vi "getEvents.vi"(8 "error in (no error)":errorcluster, 11 "ScriptEdEvents in":refnum<class "ScriptEdEvents.lvclass">) -> (0 "error out":errorcluster, 1 "eventsToScriptEd":T1, 2 "ScriptEvent":refnum<user-event>, 3 "ScriptEdEvents out":refnum<class "ScriptEdEvents.lvclass">)   [LabVIEW 2009, in "Views.lvlib" / "ScriptEditor.lvlib" / "ScriptEdEvents.lvclass"]
uses:
  ScriptEdEvents.lvclass
  ScriptEdEvents.lvclass/ScriptEdEvents.ctl
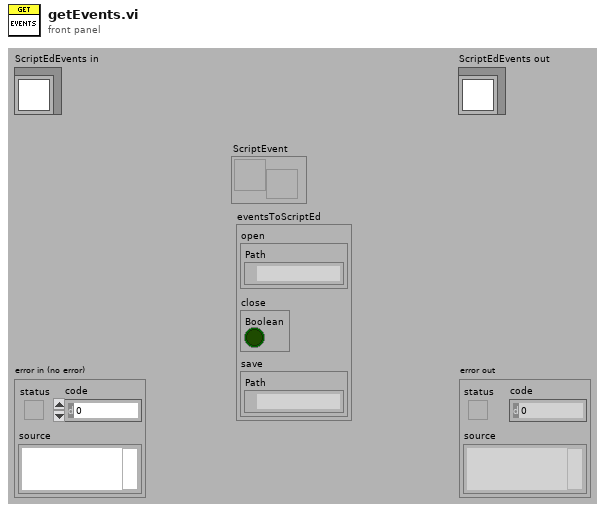
[diagram p1: front panel]
types:
  T1 = cluster{"open":cluster{"Path":path}, "close":cluster{"Boolean":bool}, "save":cluster{"Path":path}}
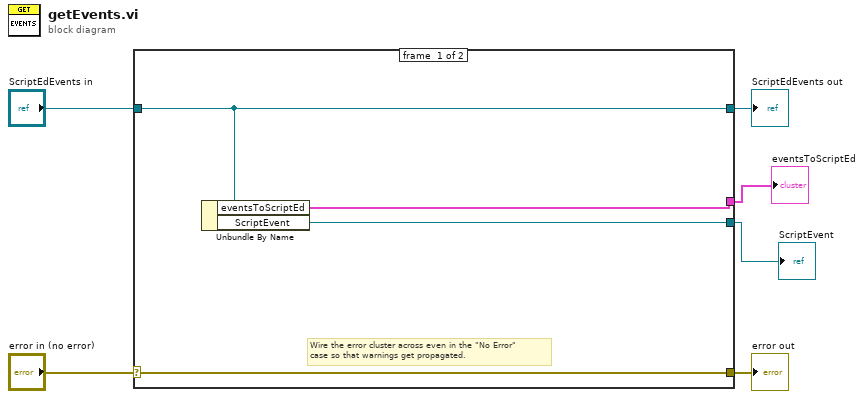
[diagram p0: block diagram]
diagram:
  n1 = case shown="No Error" "error in (no error)" {
    selector: "error in (no error)" -> [w10 w12]
    tunnel: [w10 w12] -> w5
    tunnel: [w9 w11] -> w3
    tunnel: "ScriptEdEvents in" -> [w9 w11]
    tunnel: [w8 _] -> w1
    tunnel: [w7 _] -> w2
    frame #0 {
      # "Wire the error cluster across even in the \"No Error\"\ncase so that warnings get propagated."
      n2 = Unbundle By Name(w9) -> ("eventsToScriptEd"=w7:T1, "ScriptEvent"=w8:refnum<user-event>)
    }
    frame #1 {
    }
  }
  "error out" <- w5
  "ScriptEdEvents out" <- w3
  "eventsToScriptEd" <- w2
  "ScriptEvent" <- w1
